vi "Unregister Mouse Down.vi"(8 "error in (no error)":errorcluster, 11 "UI Controller in":refnum<class "UI Controller.lvclass">) -> (0 "error out":errorcluster, 3 "UI Controller out":refnum<class "UI Controller.lvclass">)   [LabVIEW 2020, in "UI Controller.lvlib" / "UI Controller.lvclass"]
uses:
  UI Controller.lvclass
  C:/Program Files/National Instruments/LabVIEW 2020/vi.lib/ActorFrameworkMVC/Abstract Controller/Abstract Controller/Abstract Controller.lvclass
  Views/Map View/Map View Messages/Unregister Mouse Down Msg/Unregister Mouse Down Msg.lvclass
  C:/Program Files/National Instruments/LabVIEW 2020/vi.lib/ActorFramework/Message/Message.lvclass
  <vilib>/ActorFramework/Message Enqueuer/Message Enqueuer.lvclass/Message Enqueuer.ctl
  <vilib>/ActorFramework/Message Priority Queue/Priority Enqueue.vi
  <vilib>/ActorFramework/Message Enqueuer/Message Enqueuer.lvclass
  <vilib>/ActorFrameworkMVC/Abstract Controller/Abstract Controller/Abstract Controller.lvclass
panel:
  # "NOTICE -- YOU MUST LEAVE THIS NOTICE IN PLACE.\n\nCopyright (c) 2017, LIANG LIU Shawn.Liu.cn@gmail.com\nAll rights reserved.\n\nRedistribution and use in source and binary forms, with or without modification, are permitted provided that the following conditions are met:\n-Redistributions of source code must retain the above copyright notice, this list of conditions and the following disclaimer.\n-Redistributions in binary form must reproduce the above copyright notice, this list of conditions and the following disclaimer in the documentation and/or other materials provided with the distribution.\n-Neither the name of the eLp nor the names of its contributors may be used to endorse or promote products derived from this software without specific prior written permission.\n\nTHIS SOFTWARE IS PROVIDED BY THE COPYRIGHT HOLDERS AND CONTRIBUTORS \"AS IS\" AND ANY EXPRESS OR IMPLIED WARRANTIES, INCLUDING, BUT NOT LIMITED TO, THE IMPLIED WARRANTIES OF MERCHANTABILITY AND FITNESS FOR A PARTICULAR PURPOSE ARE DISCLAIMED. IN NO EVENT SHALL THE COPYRIGHT HOLDER OR CONTRIBUTORS BE LIABLE FOR ANY DIRECT, INDIRECT, INCIDENTAL, SPECIAL, EXEMPLARY, OR CONSEQUENTIAL DAMAGES (INCLUDING, BUT NOT LIMITED TO, PROCUREMENT OF SUBSTITUTE GOODS OR SERVICES; LOSS OF USE, DATA, OR PROFITS; OR BUSINESS INTERRUPTION) HOWEVER CAUSED AND ON ANY THEORY OF LIABILITY, WHETHER IN CONTRACT, STRICT LIABILITY, OR TORT (INCLUDING NEGLIGENCE OR OTHERWISE) ARISING IN ANY WAY OUT OF THE USE OF THIS SOFTWARE, EVEN IF ADVISED OF THE POSSIBILITY OF SUCH DAMAGE."
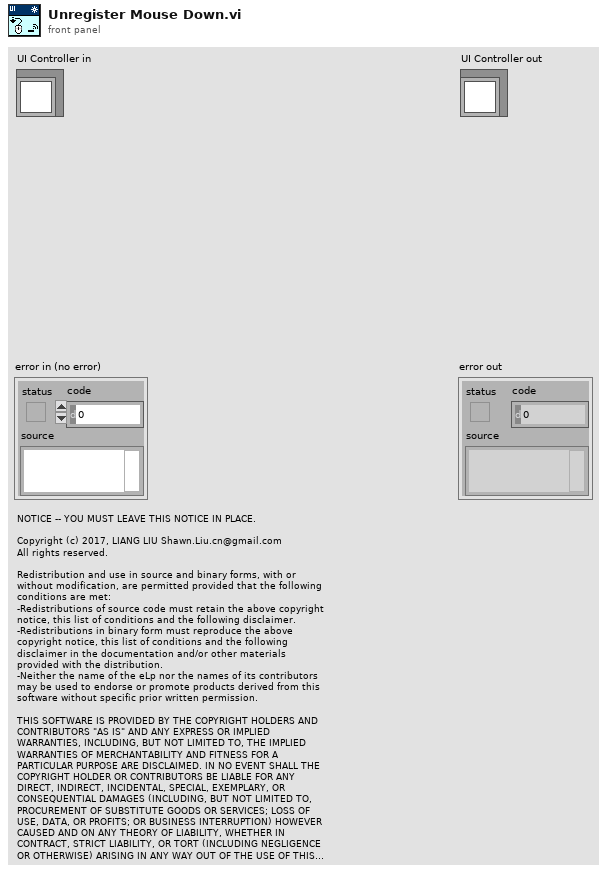
[diagram p1: front panel]
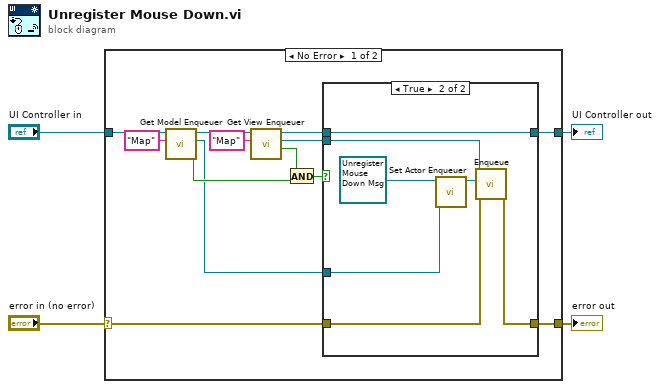
[diagram p0: block diagram]
diagram:
  n1 = case shown="No Error" "error in (no error)" {
    selector: "error in (no error)" -> [w15 w28]
    tunnel: "UI Controller in" -> [w17 w27]
    tunnel: [w16 w27] -> w3
    tunnel: [w14 w28] -> w1
    frame No Error {
      n2 = call <vilib>:"Get Model Enqueuer.vi"("Model Name"="Map", "Abstract Controller in"=w17) -> ("Found?"=w6:bool, "Model Enqueuer"=w5:refnum<class "Message Enqueuer.lvclass">, "Abstract Controller out"=w10:refnum<class "UI Controller.lvclass">)  [unwired: 6 in, 1 out]
      n3 = call <vilib>:"Get View Enqueuer.vi"("View Name"="Map", "Abstract Controller in"=w10) -> ("Found?"=w7:bool, "View Enqueuer"=w12:refnum<class "Message Enqueuer.lvclass">, "Abstract Controller out"=w11:refnum<class "UI Controller.lvclass">)  [unwired: 6 in, 1 out]
      n4 = And(x=w7, y=w6) -> (x .and. y?=w8:bool)
      n5 = case shown="True" w8 {
        tunnel: w12 -> [_ w25]
        tunnel: w11 -> [w19 w26]
        tunnel: [w19 w26] -> w16
        tunnel: w15 -> [w18 w23]
        tunnel: [w18 w22] -> w14
        tunnel: w5 -> [_ w21]
        frame False {
        }
        frame True {
          n6 = call-dynamic "Set Actor Enqueuer.vi"("Actor Enqueuer"=w21, "Unregistration Message in"=refnum<class "Unregister Mouse Down Msg.lvclass"> refnum ("Map View.lvlib:Unregister Mouse Down Msg.lvclass")) -> ("Unregistration Message out"=w24:refnum<class "Unregister Mouse Down Msg.lvclass">)  [unwired: 9 in]
          n7 = call <vilib>:"Enqueue.vi"("error in (no error)"=w23, "Message"=w24, "Message Enqueuer in"=w25) -> ("error out"=w22:errorcluster)  [unwired: 7 in, 1 out]
        }
      }
    }
    frame Error {
    }
  }
  "error out" <- w1
  "UI Controller out" <- w3
